vi "prepare dark model.vi"(8 "error in (no error)":errorcluster, 11 "Settings in":T1) -> (0 "error out":errorcluster)   [LabVIEW 2013]
uses:
  Settings/Settings.ctl
  Acquisition/Hardware Configuration.ctl
  Libraries/AS-5216-DLL/AVS settings.ctl
  Acquisition/Sphere Indicator.ctl
  Settings/Measurement Type.ctl
  Logging/Logging Configuration.ctl
  <vilib>/Analysis/baseanly.llb/Mean (DBL).vi
  <vilib>/Utility/file.llb/Write To Spreadsheet File (DBL).vi
  <vilib>/Analysis/NI_AALPro.lvlib
  <vilib>/Analysis/NI_AALBase.lvlib
  Settings/AvaSpec Settings.lvlib
  AvaSpec.lvlib
  Acquisition/AvaSpec Acquisition.lvlib
  Logging/AvaSpec Logging.lvlib
panel:
  out "Intercept Fit Verification":cluster{dbl[], "Best Power Fit":dbl[]}[](graph)
  out "Slope Fit Verification":cluster{dbl[], "Best Power Fit":dbl[]}[](graph)
  out "Offset Power model":dbl[](array[numeric])
  out "Slope Power model":dbl[](array[numeric])
  out "Average Residuals":dbl[](array[numeric])
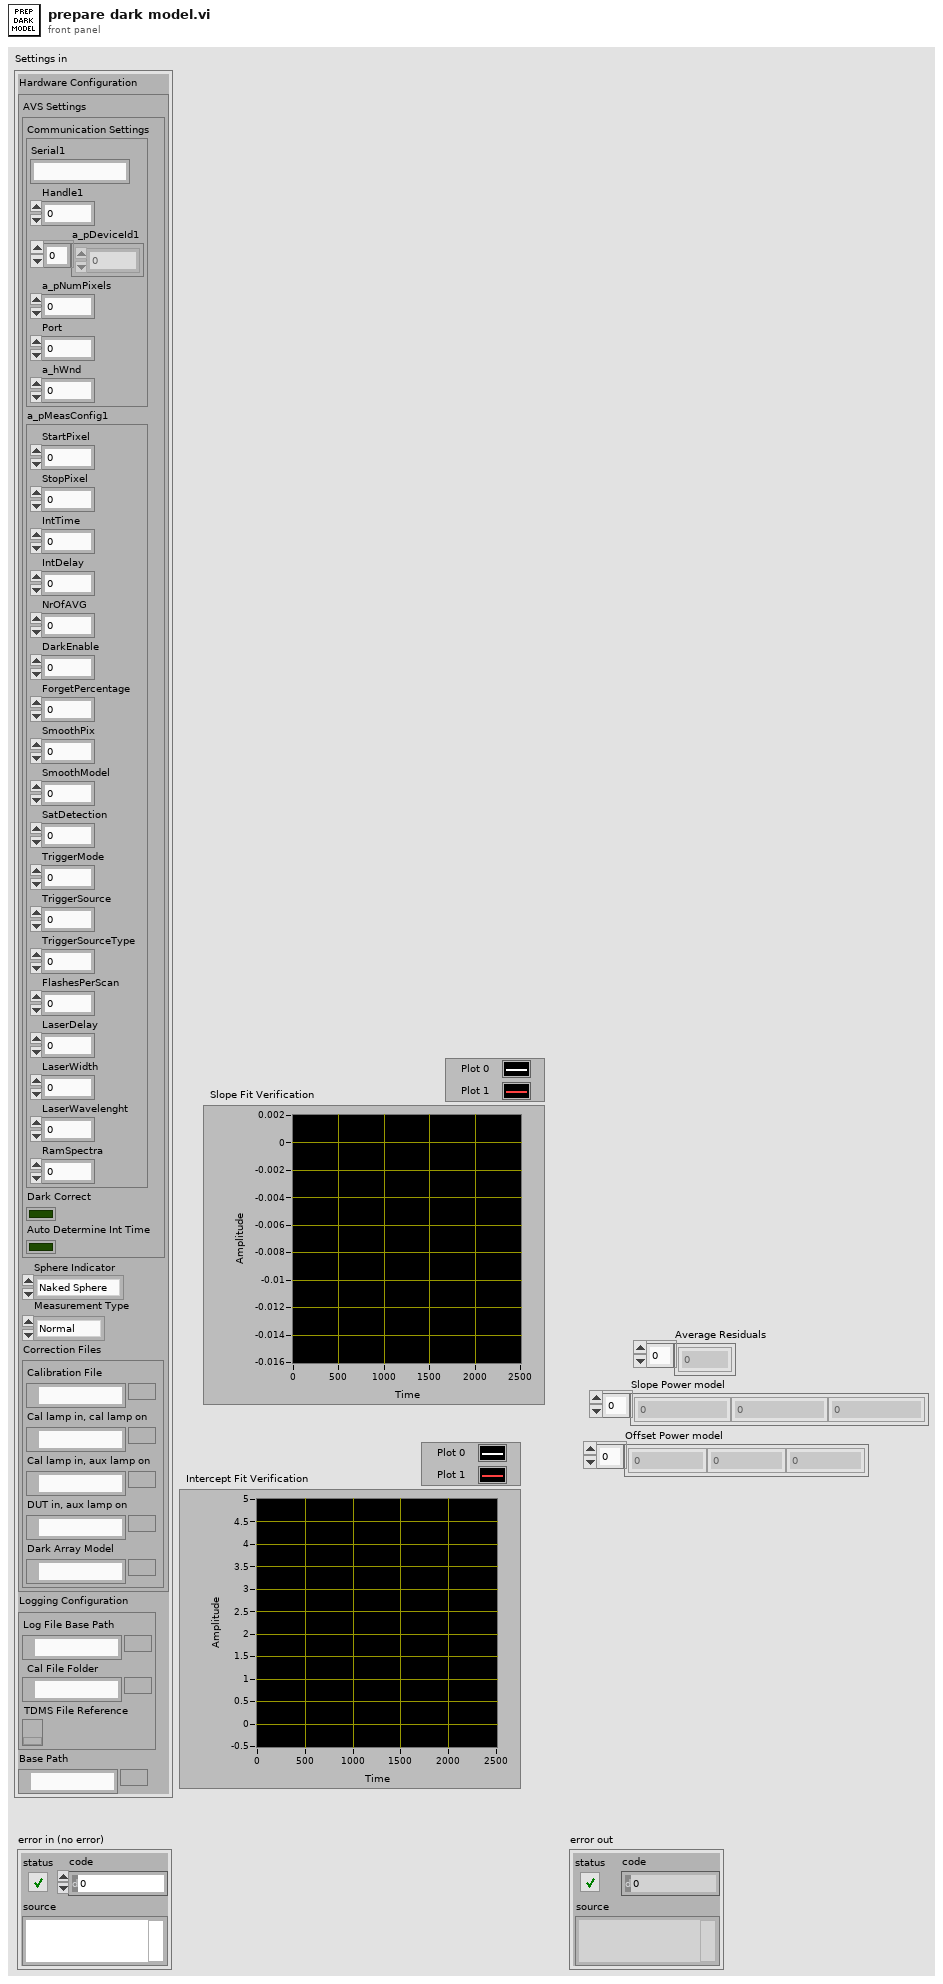
[diagram p1: front panel]
types:
  T1 = typedef "AvaSpec.lvlib/AvaSpec Settings.lvlib/Settings.ctl" = cluster{"Hardware Configuration":T2, "Logging Configuration":T6, "Base Path":path}
  T2 = typedef "AvaSpec.lvlib/AvaSpec Acquisition.lvlib/Hardware Configuration.ctl" = cluster{"AVS Settings":T3, "Sphere Indicator":T4, "Measurement Type":T5, "Correction Files":cluster{"Calibration File":path, "Cal lamp in, cal lamp on":path, "Cal lamp in, aux lamp on":path, "DUT in, aux lamp on":path, "Dark Array Model":path}}
  T3 = typedef "AvaSpec.lvlib/AVS settings.ctl" = cluster{"Communication Settings":cluster{"Serial1":string, "Handle1":i32, "a_pDeviceId1":u8[], "a_pNumPixels":u16, "Port":i32, "a_hWnd":i32}, "a_pMeasConfig1":cluster{"StartPixel":u16, "StopPixel":u16, "IntTime":sgl, "IntDelay":u32, "NrOfAVG":u32, "DarkEnable":u8, "ForgetPercentage":u8, "SmoothPix":u16, "SmoothModel":u8, "SatDetection":u8, "TriggerMode":u8, "TriggerSource":u8, "TriggerSourceType":u8, "FlashesPerScan":u16, "LaserDelay":u32, "LaserWidth":u32, "LaserWavelenght":sgl, "RamSpectra":u16}, "Dark Correct":bool, "Auto Determine Int Time":bool}
  T4 = typedef "AvaSpec.lvlib/Sphere Indicator.ctl" = enum16{"Naked Sphere", "Insulated Sphere"}
  T5 = typedef "Measurement Type.ctl" = enum16{"Normal", "Calibration", "Dark"}
  T6 = typedef "AvaSpec.lvlib/AvaSpec Logging.lvlib/Logging Configuration.ctl" = cluster{"Log File Base Path":path, "Cal File Folder":path, "TDMS File Reference":refnum<k34>}
  T7 = cluster{"amp min":dbl, "amp max":dbl, "power min":dbl, "power max":dbl, "offset min":dbl, "offset max":dbl}
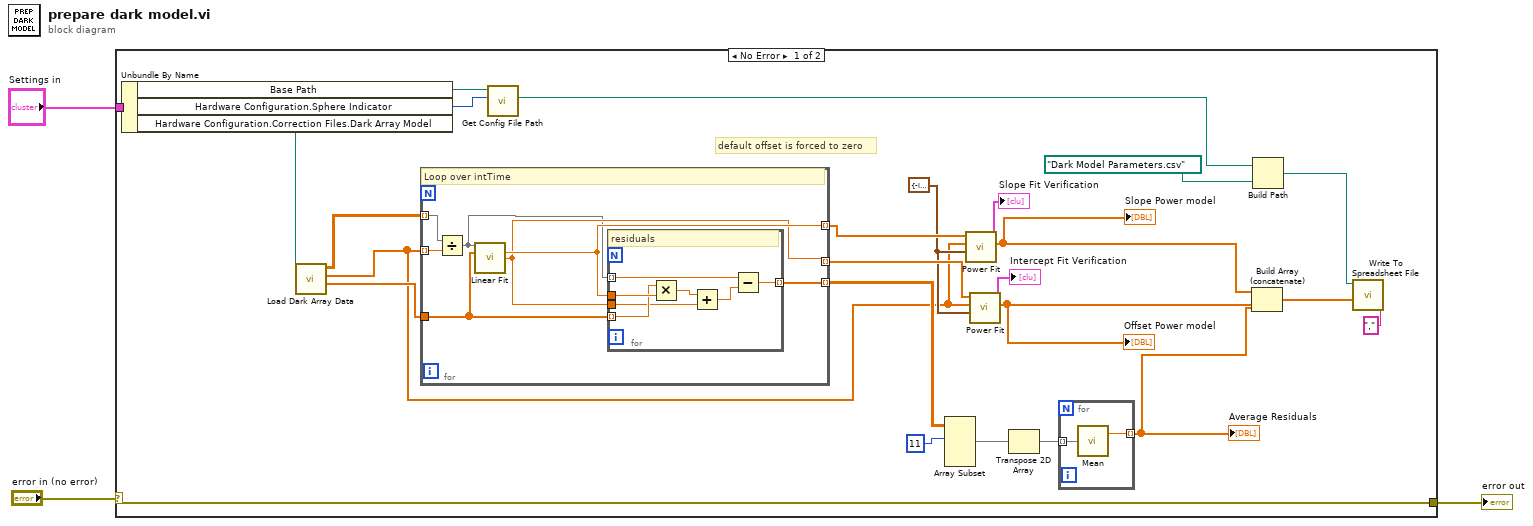
[diagram p0: block diagram]
diagram:
  n1 = case shown="No Error" "error in (no error)" {
    selector: "error in (no error)" -> [w11 w45]
    tunnel: [w11 w45] -> w2
    tunnel: "Settings in" -> [w10 _]
    frame No Error {
      w15 = T7 {"amp min"=-inf, "amp max"=inf, "power min"=-inf, "power max"=inf, "offset min"=-10.0, "offset max"=10.0} ("parameter bounds")
      # "default offset is forced to zero"
      n2 = Unbundle By Name(w10) -> ("Base Path"=w9:path, "Hardware Configuration.Sphere Indicator"=w8:T4, "Hardware Configuration.Correction Files.Dark Array Model"=w4:path)
      n3 = call "Load Dark Array Data.vi"("Dark Array Path"=w4) -> ("Freq"=w23:dbl[], "intTime"=w12:dbl[], "Scans"=w28:dbl[][])  [unwired: 8 in]
      n4 = for {
        tunnel: w28 -> [w34] mode=indexing
        tunnel: w12 -> [w32] mode=indexing
        tunnel: w23 -> [w37]
        tunnel: [w36] -> w22 mode=indexing
        tunnel: [w35] -> w16 mode=indexing
        tunnel: [w33] -> w27 mode=indexing
        # "Loop over intTime"
        n5 = Divide(x=w34, y=w32) -> (x/y=w31:dbl[])
        n6 = call <vilib>:"Linear Fit.vi"("Y"=w31, "X"=w37) -> ("slope"=w36:dbl, "intercept"=w35:dbl)  [unwired: 9 in, 3 out]
        n7 = for {
          tunnel: w37 -> [w43] mode=indexing
          tunnel: w36 -> [w44]
          tunnel: w35 -> [w41]
          tunnel: w31 -> [w39] mode=indexing
          tunnel: [w38] -> w33 mode=indexing
          # "residuals"
          n8 = Multiply(x=w43, y=w44) -> (x*y=w42:dbl)
          n9 = Add(x=w42, y=w41) -> (x+y=w40:dbl)
          n10 = Subtract(x=w39, y=w40) -> (x-y=w38:dbl)
        }
      }
      n11 = call "Get Config File Path.vi"("Sphere indicator"=w8, "Base Path"=w9) -> ("Cal File Folder"=w7:path)  [unwired: 7 in, 2 out]
      n12 = Array Subset(array=w27, index (row)=11 ("index")) -> (w19:dbl[][])  [unwired: 3 in]
      n13 = call "Power Fit.vi"("parameter bounds"=w15, "X"=w12, "Y"=w22) -> ("Power Model"=w26:dbl[], "Fit Verification"=→"Slope Fit Verification":cluster{dbl[], "Best Power Fit":dbl[]}[])  [unwired: 7 in]
      "Slope Power model" <- w26
      n14 = call "Power Fit.vi"("parameter bounds"=w15, "X"=w12, "Y"=w16) -> ("Power Model"=w13:dbl[], "Fit Verification"=→"Intercept Fit Verification":cluster{dbl[], "Best Power Fit":dbl[]}[])  [unwired: 7 in]
      "Offset Power model" <- w13
      n15 = Transpose 2D Array(2D array=w19) -> (transposed array=w18:dbl[][])
      n16 = for {
        tunnel: w18 -> [w30] mode=indexing
        tunnel: [w29] -> w17 mode=indexing
        n17 = call-poly <vilib>:"Mean.vi"("X"=w30) -> ("mean"=w29:dbl)  [unwired: 1 out]
      }
      "Average Residuals" <- w17
      n18 = Build Array (concatenate)(w26, w13, w17) -> (w25:dbl[])
      n19 = Build Path(base path=w7, name or relative path=path "Dark Model Parameters.csv" ("file path (dialog if empty)")) -> (appended path=w6:path)
      n20 = call-poly <vilib>:"Write To Spreadsheet File.vi"("delimiter (\\t)"="," ("delimiter (\\t)"), "1D data"=w25, "file path (dialog if empty)"=w6) -> ()  [unwired: 5 in, 1 out]
    }
    frame Error {
    }
  }
  "error out" <- w2
